vi "encoder_test_3mode_v0.vi"() -> ()   [LabVIEW 2014]
uses:
  <vilib>/eio/EIONode/EIONode.xnode
  <vilib>/rvi/FXPMathLib/FxpMul/XNode/nifxpmath_Multiplier.xnode
  <vilib>/rvi/FXPMathLib/sim/FxpSim.dll
  <vilib>/rvi/eio/common/nirviEmuTemplateMethod_errors.vi
  <vilib>/rvi/FXPMathLib/FxpSinAndCos/XNode/nifxpmath_SinAndCos.xnode
  <vilib>/rvi/FXPMathLib/FxpSinAndCos/simVIs/DllFxpSinAndCosTemp_sub.vi
  <vilib>/rvi/FXPMathLib/FxpSinAndCos/subVIs/nifxpmath_SinAndCos_SimConfig.ctl
  <vilib>/rvi/Analysis/measure/butterworth/XNode/niFpgaButterworthFilter.xnode
  <vilib>/rvi/FXPMathLib/FxpSub/XNode/nifxpmath_Sub.xnode
  <vilib>/rvi/FXPMathLib/FxpAdd/XNode/nifxpmath_Add.xnode
  <vilib>/rvi/DataTransferAndStorage/Container/XNode/niFpgaContainer.xnode
  <vilib>/rvi/interface/RandomDataEmulation/nirviRandomDataFpgaMultiElementTemplate.vi
panel:
  out "Dsin":fxp<+/-,28,11>
  out "Dsin_d":fxp<+/-,64,16>
  out "Dsin_dd":fxp<+/-,64,25>
  out "Sin omega":fxp<+/-,41,8>
  in  "Sin offset":fxp<+/-,27,10>
  in  "Sin magnitude":fxp<+/-,11,8>
  in  "Sin wave frequency (Hz)":fxp<+/-,21,5>
  out "Time now (s)":fxp<+,52,14>
  out "Dr":fxp<+/-,11,7> format="%.7g"
  in  "D_end":fxp<+/-,11,7>
  in  "Command type":i16(ring) items=["Step", "Ramp", "Sine"]
  out "D_i":fxp<+/-,34,18>
  in  "D_tolorence":fxp<+/-,14,3>
  in  "Ki":fxp<+/-,20,6>
  out "D_error":fxp<+/-,24,11>
  in  "Direction":bool
  out "Fmr_PD":fxp<+/-,64,31>
  in  "Kd":fxp<+/-,20,8>
  in  "Kp":fxp<+/-,20,12>
  in  "scaled coefficients_D_dd":i32[](array[numeric])=[780119100, 146811362]
  out "D_dd":fxp<+/-,36,29>
  in  "Ini coe.":bool
  out "va":fxp<+/-,38,8>
  out "vb":fxp<+/-,38,8>
  in  "stop motor":bool
  out "vq_F":fxp<+/-,20,5> format="%.57g"
  out "vd_F":fxp<+/-,20,5>
  out "D_d (mm/s)":fxp<+/-,32,12>
  out "mt":u32
  out "omega (rad/s)":fxp<+/-,32,18>
  in  "mt0":u32
  out "D(mm)":fxp<+/-,22,7>
  out "rad(NrTheta)":fxp<+/-,33,18>
  out "Encoder Position":i32
  in  "Encoder Reset":bool
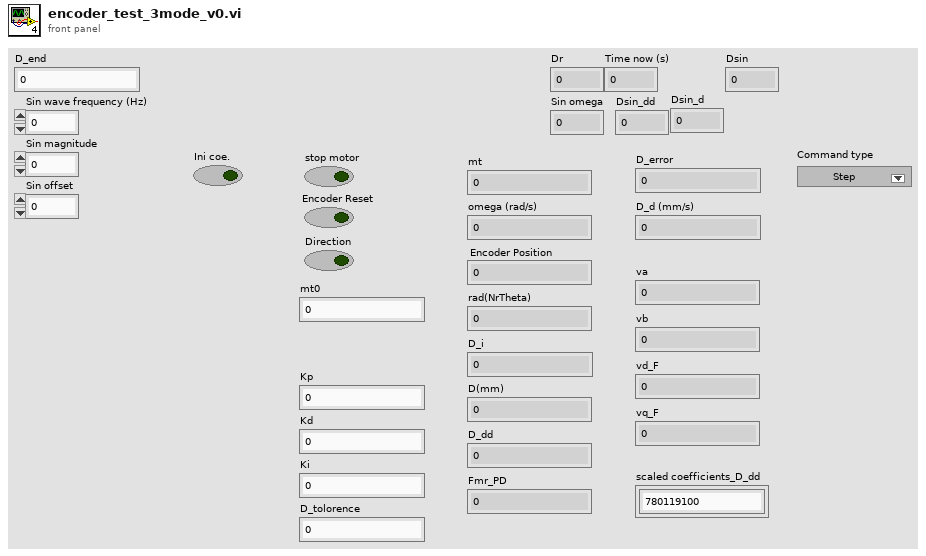
[diagram p1: front panel]
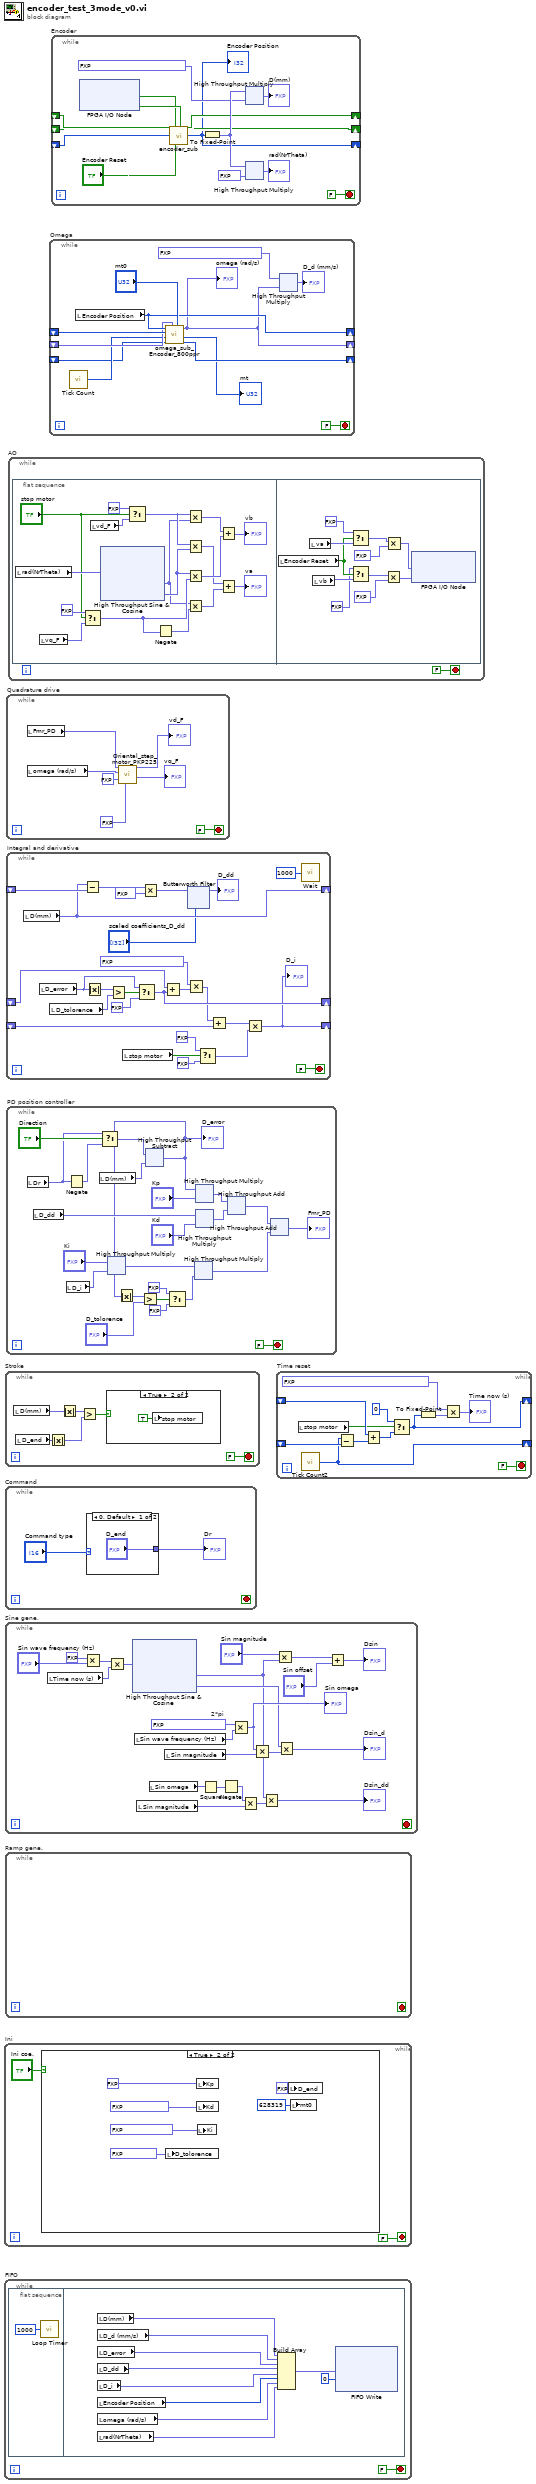
[diagram p0: block diagram]
diagram:
  n1 = while "Ini" {
    stop <- FALSE stop-if-true
    n2 = case shown="True" "Ini coe." {
      frame False {
      }
      frame True {
        n3 = local write "D_tolorence"(fxp<+/-,14,3> 0.009765625 ("D_tolorence")) -> ()
        n4 = local write "Kp"(fxp<+/-,20,12> 2.0 ("Kp")) -> ()
        n5 = local write "Kd"(fxp<+/-,20,8> 1.800048828125 ("Kd")) -> ()
        n6 = local write "Ki"(fxp<+/-,20,6> 0.0999755859375 ("D_i")) -> ()
        n7 = local write "D_end"(fxp<+/-,11,7> 20.0 ("Fmr")) -> ()
        n8 = local write "mt0"(u32 628319 ("mt0")) -> ()
      }
    }
  }
  n9 = while "FIFO" {
    stop <- FALSE stop-if-true
    n10 = flat-sequence {
      frame #0 {
        n11 = call "Loop Timer"("Count(uSec)"=u32 1000) -> ()  [unwired: 1 out]
      }
      frame #1 {
        n12 = local read "D(mm)"() -> (w18:fxp<+/-,22,7>)
        n13 = local read "D_d (mm/s)"() -> (w17:fxp<+/-,32,12>)
        n14 = local read "D_error"() -> (w16:fxp<+/-,24,11>)
        n15 = local read "D_dd"() -> (w15:fxp<+/-,36,29>)
        n16 = local read "D_i"() -> (w14:fxp<+/-,34,18>)
        n17 = local read "Encoder Position"() -> (w13:i32)
        n18 = local read "omega (rad/s)"() -> (w12:fxp<+/-,32,18>)
        n19 = local read "rad(NrTheta)"() -> (w11:fxp<+/-,33,18>)
        n20 = Build Array(w18, w17, w16, w15, w14, w13, w12, w11) -> (w19:fxp<+/-,52,32>[])
        n21 = xnode ("FIFO Write")("Element"=w19, "Timeout"=0) -> ()  [unwired: 1 in, 2 out]
      }
    }
  }
  n22 = while "Stroke" {
    stop <- FALSE stop-if-true
    n23 = local read "D(mm)"() -> (w26:fxp<+/-,22,7>)
    n24 = local read "D_end"() -> (w22:fxp<+/-,11,7>)
    n25 = Absolute Value(x=w22) -> (abs(x)=w21:fxp<+,11,7>)
    n26 = Absolute Value(x=w26) -> (abs(x)=w25:fxp<+,22,7>)
    n27 = Greater?(x=w25, y=w21) -> (0:w24:bool)
    n28 = case shown="True" w24 {
      frame False {
      }
      frame True {
        n29 = local write "stop motor"(TRUE ("stop motor")) -> ()
      }
    }
  }
  n30 = while "Command" {
    stop <- _ stop-if-true
    n31 = case shown="0, Default" "Command type" {
      tunnel: ["D_end" _] -> w28
      frame 0, Default {
      }
      frame 1 {
      }
    }
    "Dr" <- w28
  }
  n32 = while "Sine gene." {
    stop <- _ stop-if-true
    w47 = fxp<+,20,3> 6.2831878662109375  # 2*pi
    n33 = local read "Time now (s)"() -> (w50:fxp<+,52,14>)
    n34 = Multiply(x=fxp<+,1,2> 2.0, y="Sin wave frequency (Hz)") -> (x*y=w51:fxp<+/-,21,6>)
    n35 = Multiply(x=w51, y=w50) -> (x*y=w31:fxp<+/-,64,20>)
    n36 = xnode "High Throughput Sine & Cosine"("x (pi)"=w31) -> ("sin(x)"=w35:fxp<+/-,16,2>, "cos(x)"=w42:fxp<+/-,16,2>)
    n37 = local read "Sin wave frequency (Hz)"() -> (w46:fxp<+/-,21,5>)
    n38 = local read "Sin magnitude"() -> (w37:fxp<+/-,11,8>)
    n39 = local read "Sin omega"() -> (w38:fxp<+/-,41,8>)
    n40 = local read "Sin magnitude"() -> (w41:fxp<+/-,11,8>)
    n41 = Square(x=w38) -> (x^2=w39:fxp<+,64,14>)
    n42 = Negate(x=w39) -> (-x=w36:fxp<+/-,64,15>)
    n43 = Multiply(x=w47, y=w46) -> (x*y=w43:fxp<+/-,41,8>)
    "Sin omega" <- w43
    n44 = Multiply(x=w36, y=w37) -> (x*y=w40:fxp<+/-,64,23>)
    n45 = Multiply(x=w43, y=w41) -> (x*y=w48:fxp<+/-,51,15>)
    n46 = Multiply(x=w35, y=w40) -> (x*y=→"Dsin_dd":fxp<+/-,64,25>)
    n47 = Multiply(x="Sin magnitude", y=w35) -> (x*y=w49:fxp<+/-,27,10>)
    n48 = Multiply(x=w42, y=w48) -> (x*y=→"Dsin_d":fxp<+/-,64,16>)
    n49 = Add(x=w49, y="Sin offset") -> (x+y=→"Dsin":fxp<+/-,28,11>)
  }
  n50 = while "Ramp gene." {
    stop <- _ stop-if-true
  }
  n51 = while "Quadrature drive" {
    stop <- FALSE stop-if-true
    n52 = local read "Fmr_PD"() -> (w84:fxp<+/-,64,31>)
    n53 = local read "omega (rad/s)"() -> (w86:fxp<+/-,32,18>)
    n54 = call "Oriental_step_motor_PKP225.vi"("F_Threshold"=fxp<+,12,12> 10.0, "dFmr"=fxp<+/-,25,15> 0.0, "omega"=w86, "Fmr"=w84) -> ("vq_F"=→"vq_F":fxp<+/-,20,5>, "vd_F"=→"vd_F":fxp<+/-,20,5>)  [unwired: 6 in]
  }
  n55 = while "Integral and derivative" {
    shift-right: [w111] -> _
    shift-left: _ -> [w115]
    shift-right: [w101] -> _
    shift-left: _ -> [w102]
    shift-right: [w91] -> _
    shift-left: _ -> [w95]
    stop <- FALSE stop-if-true
    n56 = local read "D(mm)"() -> (w111:fxp<+/-,22,7>)
    n57 = local read "D_error"() -> (w103:fxp<+/-,24,11>)
    n58 = local read "D_tolorence"() -> (w106:fxp<+/-,14,3>)
    n59 = Subtract(x=w111, y=w115) -> (x-y=w114:fxp<+/-,23,8>)
    n60 = Absolute Value(x=w103) -> (abs(x)=w107:fxp<+,24,11>)
    n61 = Greater?(x=w107, y=w106) -> (0:w105:bool)
    n62 = local read "stop motor"() -> (w98:bool)
    n63 = Select(t=w103, s=w105, f=fxp<+,24,11> 0.0) -> (s? t:f=w101:fxp<+/-,25,12>)
    n64 = Multiply(x=w114, y=fxp<+/-,33,13> 1000.0) -> (x*y=w112:fxp<+/-,55,20>)
    n65 = Add(x=w102, y=w101) -> (x+y=w100:fxp<+/-,26,13>)
    n66 = Multiply(x=fxp<+/-,30,12> 0.000499725341796875, y=w100) -> (x*y=w94:fxp<+/-,55,24>)
    n67 = xnode "Butterworth Filter"("input data"=w112, "scaled coefficients"="scaled coefficients_D_dd") -> ("output data"=→"D_dd":fxp<+/-,36,24>)  [unwired: 1 in]
    n68 = Select(t=fxp<+,1,1> 0.0, s=w98, f=fxp<+,1,1> 1.0) -> (s? t:f=w92:fxp<+,1,1>)
    n69 = Add(x=w94, y=w95) -> (x+y=w93:fxp<+/-,32,16>)
    n70 = Multiply(x=w93, y=w92) -> (x*y=w91:fxp<+/-,32,16>)
    "D_i" <- w91
    n71 = call "Wait"("Count(uSec)"=u32 1000) -> ()  [unwired: 1 out]
  }
  n72 = while "PD position controller" {
    stop <- FALSE stop-if-true
    n73 = local read "Dr"() -> (w125:fxp<+/-,11,7>)
    n74 = local read "D_dd"() -> (w144:fxp<+/-,36,29>)
    n75 = local read "D_i"() -> (w136:fxp<+/-,34,18>)
    n76 = Negate(x=w125) -> (-x=w140:fxp<+/-,12,8>)
    n77 = local read "D(mm)"() -> (w148:fxp<+/-,22,7>)
    n78 = Select(t=w125, s="Direction", f=w140) -> (s? t:f=w139:fxp<+/-,12,8>)
    n79 = xnode ("High Throughput Multiply")("x"="Ki", "y"=w136) -> ("x*y"=w130:fxp<+/-,54,24>)
    n80 = xnode "High Throughput Subtract"("x"=w139, "y"=w148) -> ("x-y"=w134:fxp<+/-,24,9>)
    "D_error" <- w134
    n81 = Absolute Value(x=w134) -> (abs(x)=w135:fxp<+,24,9>)
    n82 = Greater?(x=w135, y="D_tolorence") -> (0:w133:bool)
    n83 = Select(t=fxp<+,10,2> 1.0, s=w133, f=fxp<+,10,2> 0.0) -> (s? t:f=w129:fxp<+,10,2>)
    n84 = xnode ("High Throughput Multiply")("x"=w130, "y"=w129) -> ("x*y"=w126:fxp<+/-,64,26>)
    n85 = xnode ("High Throughput Multiply")("x"=w134, "y"="Kp") -> ("x*y"=w146:fxp<+/-,44,21>)
    n86 = xnode ("High Throughput Multiply")("x"=w144, "y"="Kd") -> ("x*y"=w145:fxp<+/-,56,37>)
    n87 = xnode ("High Throughput Add")("x"=w146, "y"=w145) -> ("x+y"=w127:fxp<+/-,61,38>)
    n88 = xnode ("High Throughput Add")("x"=w127, "y"=w126) -> ("x+y"=→"Fmr_PD":fxp<+/-,64,39>)
  }
  n89 = while "AO" {
    stop <- FALSE stop-if-true
    n90 = flat-sequence {
      frame #0 {
        n91 = local read "rad(NrTheta)"() -> (w165:fxp<+/-,33,18>)
        n92 = local read "vq_F"() -> (w163:fxp<+/-,20,5>)
        n93 = Select(t=fxp<+,20,5> 0.0, s="stop motor", f=w163) -> (s? t:f=w160:fxp<+/-,21,6>)
        n94 = local read "vd_F"() -> (w164:fxp<+/-,20,5>)
        n95 = xnode "High Throughput Sine & Cosine"("x (pi)"=w165) -> ("sin(x)"=w156:fxp<+/-,17,2>, "cos(x)"=w158:fxp<+/-,17,2>)
        n96 = Select(t=fxp<+,20,5> 0.0, s="stop motor", f=w164) -> (s? t:f=w157:fxp<+/-,21,6>)
        n97 = Negate(x=w160) -> (-x=w159:fxp<+/-,21,6>)
        n98 = Multiply(x=w157, y=w156) -> (x*y=w155:fxp<+/-,37,7>)
        n99 = Multiply(x=w157, y=w158) -> (x*y=w153:fxp<+/-,37,7>)
        n100 = Multiply(x=w158, y=w160) -> (x*y=w154:fxp<+/-,37,7>)
        n101 = Multiply(x=w156, y=w159) -> (x*y=w152:fxp<+/-,37,7>)
        n102 = Add(x=w155, y=w154) -> (x+y=→"vb":fxp<+/-,38,8>)
        n103 = Add(x=w153, y=w152) -> (x+y=→"va":fxp<+/-,38,8>)
      }
      frame #1 {
        n104 = local read "Encoder Reset"() -> (w199:bool)
        n105 = local read "va"() -> (w201:fxp<+/-,38,8>)
        n106 = local read "vb"() -> (w200:fxp<+/-,38,8>)
        n107 = Select(t=fxp<+/-,20,5> 5.0 ("y"), s=w199, f=w201) -> (s? t:f=w202:fxp<+/-,38,8>)
        n108 = Select(t=fxp<+/-,20,5> 0.0 ("y"), s=w199, f=w200) -> (s? t:f=w203:fxp<+/-,38,8>)
        n109 = Multiply(x=w203, y=fxp<+/-,20,5> -0.5) -> (x*y=w207:fxp<+/-,57,12>)
        n110 = Multiply(x=w202, y=fxp<+/-,20,5> -0.5) -> (x*y=w206:fxp<+/-,57,12>)
        n111 = xnode "FPGA I/O Node"("Mod8/AO0"=w206, "Mod8/AO1"=w207) -> ()  [unwired: 2 in, 2 out]
      }
    }
  }
  n112 = while "Omega" {
    shift-right: [w217] -> _
    shift-left: _ -> [w218]
    shift-right: [w210] -> _
    shift-left: _ -> [w216]
    shift-right: [w213] -> _
    shift-left: _ -> [w214]
    stop <- FALSE stop-if-true
    n113 = call "Tick Count"() -> ("Tick Count(Ticks)"=w215:u32)
    n114 = local read "Encoder Position"() -> (w217:i32)
    n115 = call "omega_sub_Encoder_800ppr.vi"("mt0"="mt0", "omega_pre"=w216, "ticks_m_pre"=w214, "ticks"=w215, "count_pre"=w218, "count"=w217) -> ("ticks_m"=w213:u32, "mt"=→"mt":u32, "omega"=w210:fxp<+/-,20,9>)  [unwired: 3 in]
    "omega (rad/s)" <- w210
    n116 = xnode ("High Throughput Multiply")("x"=fxp<+/-,26,1> 0.3183099031448364, "y"=w210) -> ("x*y"=→"D_d (mm/s)":fxp<+/-,46,10>)
  }
  n117 = while "Encoder" {
    shift-right: [w226] -> _
    shift-left: _ -> [w228]
    shift-right: [w225] -> _
    shift-left: _ -> [w227]
    shift-right: [w223] -> _
    shift-left: _ -> [w224]
    stop <- FALSE stop-if-true
    n118 = xnode "FPGA I/O Node"() -> ("Mod4/DI3"=w233:bool, "Mod4/DI4"=w234:bool)  [unwired: 2 in, 2 out]
    n119 = call "encoder_sub.vi"("A_pre"=w228, "B_pre"=w227, "Encoder Position_pre"=w224, "A input"=w233, "Encoder Position Reset"="Encoder Reset", "B input"=w234) -> ("A"=w226:bool, "B"=w225:bool, "Encoder Position (Counts)"=w223:i32)  [unwired: 19 in]
    "Encoder Position" <- w223
    n120 = To Fixed-Point(number=w223) -> (fixed-point=w231:fxp<+/-,32,32>)  [unwired: 1 in]
    n121 = xnode ("High Throughput Multiply")("x"=w231, "y"=fxp<+/-,24,0> 0.002499997615814209) -> ("x*y"=→"D(mm)":fxp<+/-,56,32>)
    n122 = xnode ("High Throughput Multiply")("x"=w231, "y"=fxp<+/-,24,0> 0.125) -> ("x*y"=→"rad(NrTheta)":fxp<+/-,56,32>)
  }
  n123 = while "Time reset" {
    shift-right: [w238] -> _
    shift-left: _ -> [w245]
    shift-right: [w240] -> _
    shift-left: _ -> [w241]
    stop <- FALSE stop-if-true
    n124 = local read "stop motor"() -> (w243:bool)
    n125 = call "Tick Count2"() -> ("Tick Count(uSec)"=w240:u32)
    n126 = Subtract(x=w240, y=w241) -> (x-y=w246:u32)
    n127 = Add(x=w245, y=w246) -> (x+y=w244:u32)
    n128 = Select(t=u32 0, s=w243, f=w244) -> (s? t:f=w238:u32)
    n129 = To Fixed-Point(number=w238) -> (fixed-point=w237:fxp<+,32,32>)  [unwired: 1 in]
    n130 = Multiply(x=fxp<+,20,-18> 1.0000003385357559e-06, y=w237) -> (x*y=→"Time now (s)":fxp<+,52,14>)
  }
